vi "Read Response.vi"(8 "error in":errorcluster, 11 "Luminos in":refnum<class "Luminos.lvclass">) -> (0 "error out":errorcluster, 2 "Success?":bool, 3 "Luminos out":refnum<class "Luminos.lvclass">)   [LabVIEW 2018, in "Luminos.lvlib" / "Luminos.lvclass"]
uses:
  Luminos.lvclass
  Luminos.lvclass/Luminos.ctl
  <instrlib>/ZaberTSeries/ZaberTSeries.lvlib
  PPLs/Axis/Axis.lvlibp/Axis.lvclass
  C:/Projects/LabVIEW/PPLs/Axis/Axis.lvlibp/Axis.lvclass
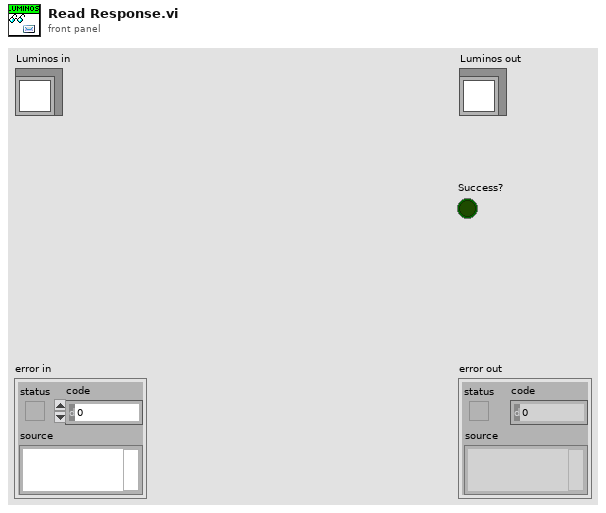
[diagram p1: front panel]
types:
  T1 = typedef "ZaberTSeries.lvlib/Response.ctl" = cluster{"Device Number":u8, "Command":u8, "Data":i32}
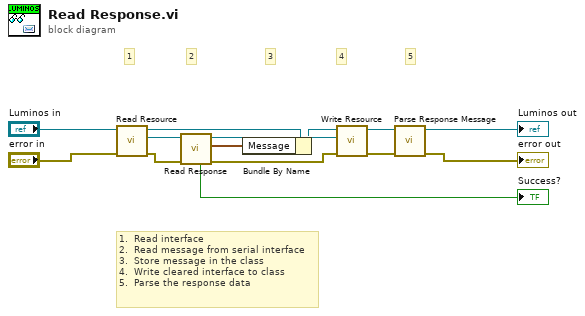
[diagram p0: block diagram]
diagram:
  # "1.  Read interface\n2.  Read message from serial interface\n3.  Store message in the class\n4.  Write cleared interface to class\n5.  Parse the response data"
  # "5"
  # "4"
  # "3"
  # "2"
  # "1"
  n1 = call "Read Resource.vi"("error in"="error in", "Axis in"="Luminos in") -> ("error out"=w8:errorcluster, "Resource"=w9:refnum<visa-resource-name>, "Axis out"=w14:refnum<class "Luminos.lvclass">)  [unwired: 7 in]
  n2 = call <instrlib>:"Read Response.vi"("error in (no error)"=w8, "VISA resource name"=w9) -> ("error out"=w12:errorcluster, "Response"=w6:T1, "VISA resource name out"=w13:refnum<visa-resource-name>, "Response Received?"=→"Success?":bool)  [unwired: 5 in, 1 out]
  n3 = Bundle By Name(cluster=w14, "Message"=w6) -> (w7:refnum<class "Luminos.lvclass">)
  n4 = call "Write Resource.vi"("error in"=w12, "Resource"=w13, "Axis in"=w7) -> ("error out"=w3:errorcluster, "Axis out"=w5:refnum<class "Luminos.lvclass">)  [unwired: 7 in]
  n5 = call-dynamic "Parse Response Message.vi"("error in"=w3, "Luminos in"=w5) -> ("error out"=→"error out":errorcluster, "Luminos out"=→"Luminos out":refnum<class "Luminos.lvclass">)  [unwired: 8 in]
